vi "GetResult&PrintLog.vi"(5 "Str引用句柄":refnum<vi>, 6 "RX标准":string, 7 "TX标准":string, 8 "RX测量":string, 9 "TX测量":string) -> (3 "布尔":bool)   [LabVIEW 2014]
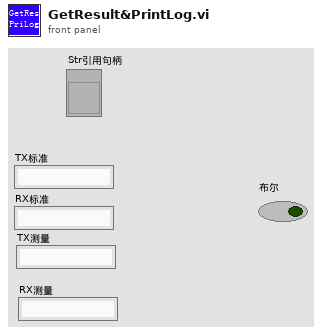
[diagram p1: front panel]
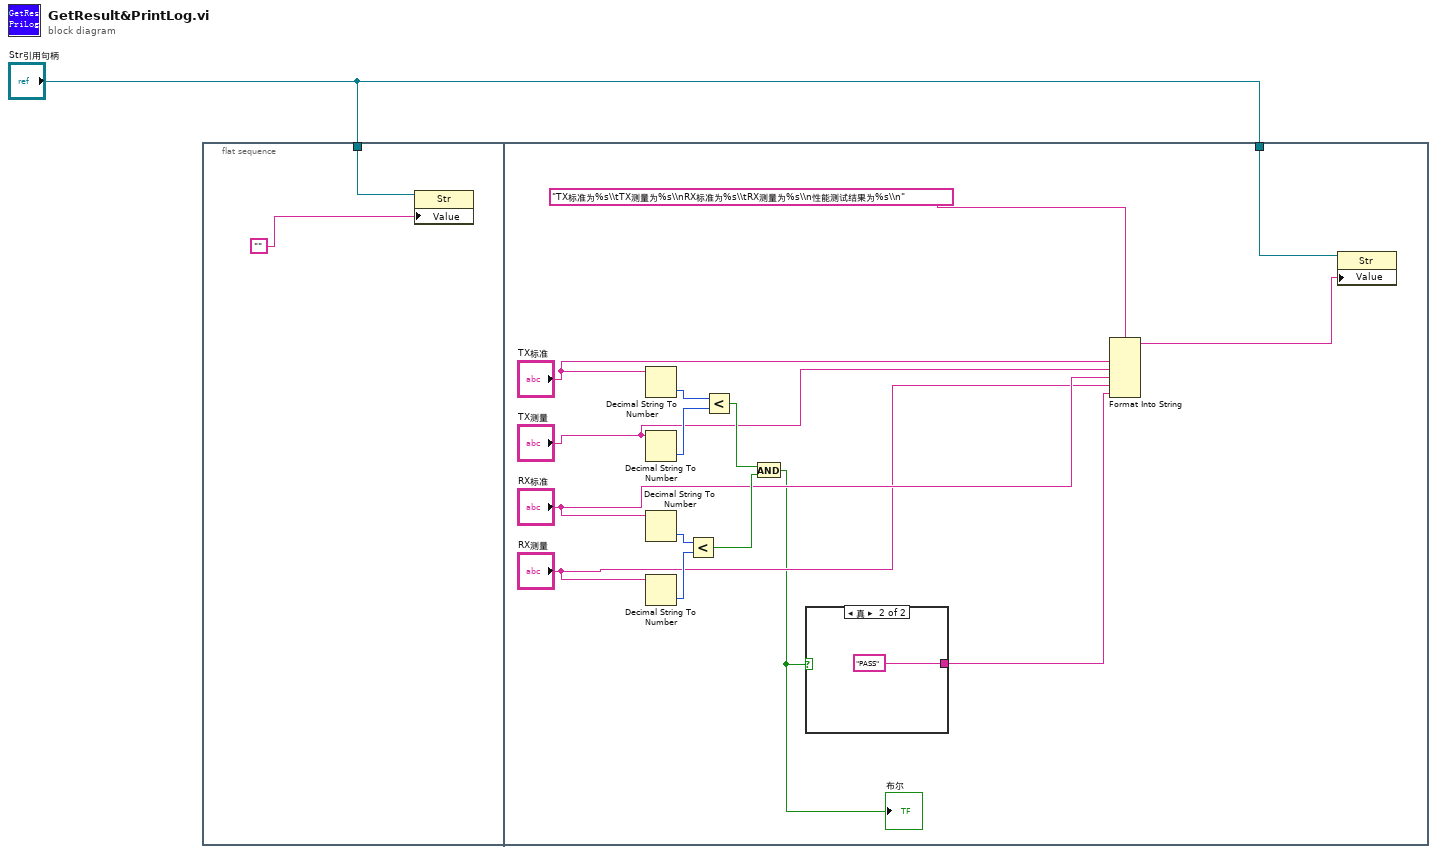
[diagram p0: block diagram]
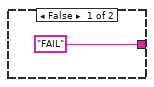
[diagram p2: hidden frame]
diagram:
  n1 = flat-sequence {
    tunnel: "Str引用句柄" -> [w3]
    tunnel: "Str引用句柄" -> [w18]
    frame #0 {
      n2 = property class="Str"(reference=w3, "Value"="") -> ()  [unwired: 1 in, 2 out]
    }
    frame #1 {
      n3 = Decimal String To Number(string="TX标准") -> (number=w17:i32)  [unwired: 2 in, 1 out]
      n4 = Decimal String To Number(string="TX测量") -> (number=w16:i32)  [unwired: 2 in, 1 out]
      n5 = Decimal String To Number(string="RX标准") -> (number=w15:i32)  [unwired: 2 in, 1 out]
      n6 = Decimal String To Number(string="RX测量") -> (number=w14:i32)  [unwired: 2 in, 1 out]
      n7 = Less?(x=w15, y=w14) -> (x < y?=w12:bool)
      n8 = Less?(x=w17, y=w16) -> (x < y?=w13:bool)
      n9 = And(x=w13, y=w12) -> (x .and. y?=w4:bool)
      "布尔" <- w4
      n10 = case shown="真" w4 {
        tunnel: ["FAIL" "PASS"] -> w6
        frame False {
        }
        frame True {
        }
      }
      n11 = Format Into String(format string="TX标准为%s\\tTX测量为%s\\nRX标准为%s\\tRX测量为%s\\n性能测试结果为%s\\n", "TX标准", "TX测量", "RX标准", "RX测量", w6) -> (resulting string=w5:string)  [unwired: 2 in, 1 out]
      n12 = property class="Str"(reference=w18, "Value"=w5) -> ()  [unwired: 1 in, 2 out]
    }
  }
